vi "emi_Get VI Revision in non Real Time.vi"(0 "VI Refnum(This VI)":refnum<vi>, 11 "error in (no error)":errorcluster) -> (4 "VI Refnum Out":refnum<vi>, 8 "Vi rev. no":u32, 15 "error out":errorcluster)   [LabVIEW 2011]
doc: "Return the VI revision when in development mode, for window targets."
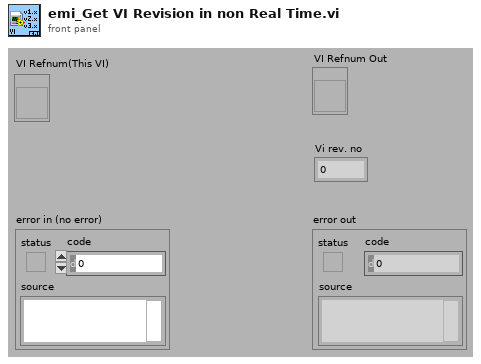
[diagram p1: front panel]
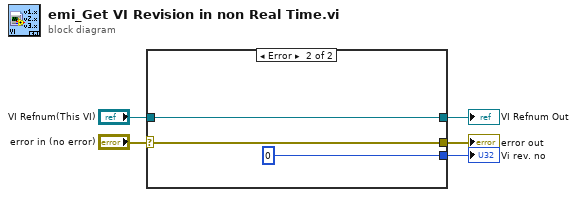
[diagram p0: block diagram]
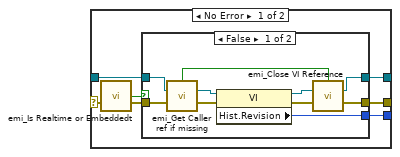
[diagram p2: hidden frame]
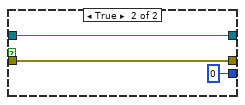
[diagram p3: hidden frame]
diagram:
  n1 = case shown="Error" "error in (no error)" {
    selector: "error in (no error)" -> [w8 w27]
    tunnel: "VI Refnum(This VI)" -> [w9 w28]
    tunnel: [w10 w28] -> w4
    tunnel: [w12 u32 0 ("Hist.Revision")] -> w3
    tunnel: [w11 w27] -> w2
    frame No Error {
      n2 = call "emi_Is Realtime or Embeddedt.vi"("error in (no error)"=w8) -> ("RT||Emb?"=w7:bool, "error out"=w6:errorcluster)  [unwired: 13 in]
      n3 = case shown="False" w7 {
        tunnel: [w21 u32 0 ("Hist.Revision")] -> w12
        tunnel: [w19 w24] -> w11
        tunnel: [w18 w23] -> w10
        tunnel: w6 -> [w15 w24]
        tunnel: w9 -> [w14 w23]
        frame False {
          n4 = call "emi_Get Caller ref if missing.vi"("VI Refnum(Calling VI)"=w14, "error in (no error)"=w15) -> ("Ref Generated"=w22:bool, "VI Refnum Out"=w13:refnum<vi>, "error out"=w16:errorcluster)  [unwired: 11 in]
          n5 = property class="VI"(reference=w13, error in=w16) -> (reference out=w17:refnum<vi>, error out=w20:errorcluster, "Hist.Revision"=w21:u32)
          n6 = call "emi_Close VI Reference.vi"("Close ref?(T)"=w22, "VI Refnum"=w17, "error in (no error)"=w20) -> ("VI Refnum Out"=w18:refnum<vi>, "error out"=w19:errorcluster)  [unwired: 11 in]
        }
        frame True {
        }
      }
    }
    frame Error {
    }
  }
  "VI Refnum Out" <- w4
  "Vi rev. no" <- w3
  "error out" <- w2
